vi "Return_Gauge_SubVi.vi"(11 "stop":bool) -> (3 "Numeric":i32)   [LabVIEW 2014]
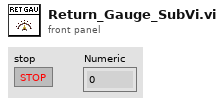
[diagram p1: front panel]
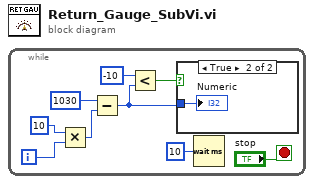
[diagram p0: block diagram]
diagram:
  n1 = while {
    i -> [w9]
    stop <- "stop" stop-if-true
    n2 = Multiply(x=10, y=w9) -> (x*y=w7:i32)
    n3 = Subtract(x=1030, y=w7) -> (x-y=w4:i32)
    n4 = Less?(x=-10, y=w4) -> (x < y?=w2:bool)
    n5 = case shown="True" w2 {
      tunnel: w4 -> [_ w10]
      frame False {
      }
      frame True {
        "Numeric" <- w10
      }
    }
    n6 = Wait (ms)(milliseconds to wait=u32 10) -> ()  [unwired: 1 out]
  }
